vi "SCC Undo Check Out.vi"(7 "advanced options":variant, 8 "error in (no error)":errorcluster, 10 "files":path[](array[path]), 11 "source control reference in":T1) -> (0 "error out":errorcluster, 1 "dialog box cancelled?":bool, 2 "status message":string, 3 "source control reference out":T1)   [LabVIEW 2017, in "NI_SCC.lvlib"]
doc: "Cancels a previous source control check-out operation and restores the contents of the selected file to the previous version. Any changes you made to the file are lost."
uses:
  <vilib>/SourceControl/sccapi/NI_SCC.lvlib
  <vilib>/SourceControl/sccapi/SCCAPI Refnum.ctl
  <vilib>/SourceControl/sccapi/SCCAPI SCC Operations.ctl
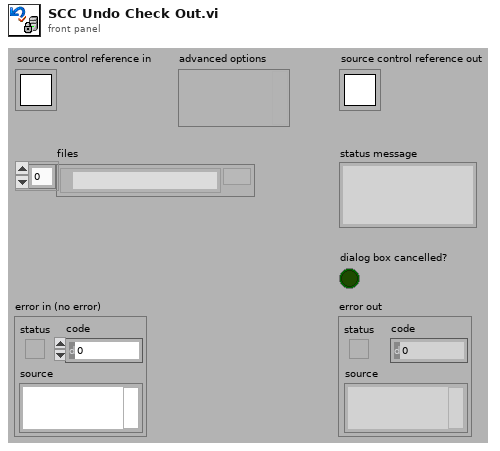
[diagram p1: front panel]
types:
  T1 = typedef "NI_SCC.lvlib/SCCAPI Refnum.ctl" = refnum<k1>
  T2 = typedef "NI_SCC.lvlib/SCCAPI SCC Operations.ctl" = enum16{"Add", "Check In", "Check Out", "Close Project", "Compare Files", "Compare VIs", "Configure Project", "File History", "File Properties", "File Status", "Find All Providers", "Get Advanced Command Options", "Get File Copy", "Get Latest Version", "Get Project Name", "Get StaticVI Path", "Initialize", "Not A Source Control Reference", "Open Project", "Provider Supports Functionality", "Remove", "Run Provider", "Undo Check Out", "Uninitialize", "Is File In Local Path"}
  T3 = typedef "SCCAPI Refnum.ctl" = refnum<k1>
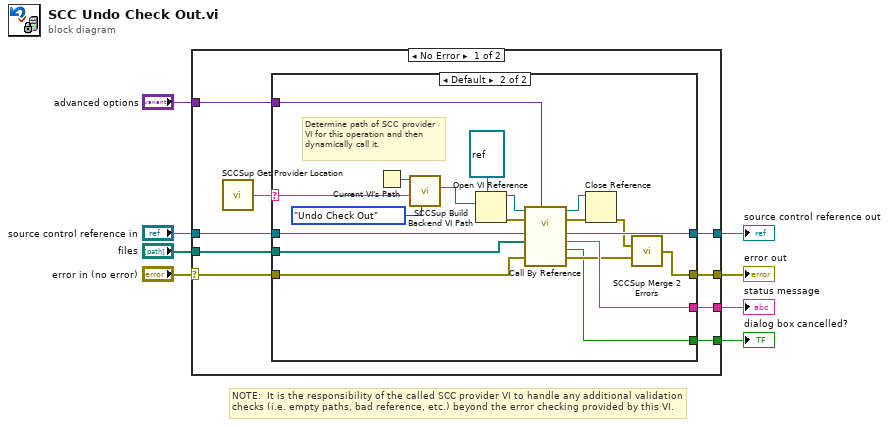
[diagram p0: block diagram]
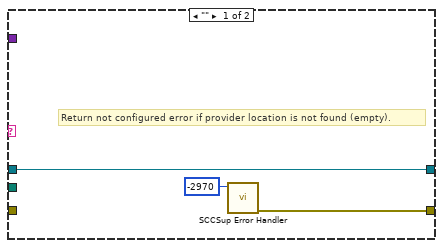
[diagram p2: hidden frame]
diagram:
  # "NOTE:  It is the responsibility of the called SCC provider VI to handle any additional validation checks (i.e. empty paths, bad reference, etc.) beyond the error checking provided by this VI."
  n1 = case shown="No Error" "error in (no error)" {
    selector: "error in (no error)" -> [w11 w41]
    tunnel: [w17 w41] -> w7
    tunnel: "source control reference in" -> [w16 w40]
    tunnel: [w15 _] -> w5
    tunnel: [w14 w40] -> w4
    tunnel: "files" -> [w13 _]
    tunnel: [w10 _] -> w2
    tunnel: "advanced options" -> [w9 _]
    frame No Error {
      n2 = call <vilib>:"SCCSup Get Provider Location.vi"() -> ("provider location"=w12:string)  [unwired: 6 in]
      n3 = case shown="Default" w12 {
        selector: w12 -> [_ w24]
        tunnel: [w18 w39] -> w17
        tunnel: w16 -> [w20 w31]
        tunnel: [_ w38] -> w15
        tunnel: [w20 w32] -> w14
        tunnel: w13 -> [_ w30]
        tunnel: w11 -> [_ w23]
        tunnel: [_ w22] -> w10
        tunnel: w9 -> [_ w21]
        frame "" {
          # "Return not configured error if provider location is not found (empty)."
          n4 = call <vilib>:"SCCSup Error Handler.vi"("scc error code"=-2970 ("code")) -> ("error out"=w18:errorcluster)  [unwired: 10 in]
        }
        frame Default {
          # "Determine path of SCC provider VI for this operation and then dynamically call it."
          n5 = Current VI's Path() -> (path=w27:path)
          n6 = call <vilib>:"SCCSup Build Backend VI Path.vi"("scc operation"=SCCAPI_SCC_Operations."Undo Check Out", "provider location"=w24, "caller path"=w27) -> ("scc backend VI path"=w26:path)  [unwired: 8 in]
          n7 = Open VI Reference(type specifier VI Refnum (for type only)=refnum<vi> refnum, vi path=w26) -> (vi reference=w36:refnum<vi>, error out=w35:errorcluster)  [unwired: 4 in]
          n8 = call-by-ref "?"(reference=w36, error in=w35, "advanced options"=w21, "error in (no error)"=w23, "files"=w30, "source control reference in"=w31) -> (reference out=w34:refnum<vi>, error out=w33:errorcluster, 0:"error out"=w28:errorcluster, "dialog box cancelled?"=w22:bool, "status message"=w38:string, "source control reference out"=w32:T3)  [unwired: 4 in]
          n9 = Close Reference(reference=w34, error in (no error)=w33) -> (error out=w29:errorcluster)
          n10 = call <vilib>:"SCCSup Merge 2 Errors.vi"("Error IO 1"=w29, "Error IO 2"=w28) -> ("Error IO out"=w39:errorcluster)  [unwired: 13 in]
        }
      }
    }
    frame Error {
    }
  }
  "error out" <- w7
  "status message" <- w5
  "source control reference out" <- w4
  "dialog box cancelled?" <- w2
